vi "Wechart Get Token.vi"(8 "error in":errorcluster, 10 "appsecret":string="f200cec5fffa0616111cce48b6bc0b68", 11 "appID":string="wx6df44cfeabb6273b") -> (0 "error out":errorcluster, 3 "Token":string)   [LabVIEW 2020]
uses:
  <vilib>/httpClient/POSTBuffer.vi
  <vilib>/httpClient/LabVIEWHTTPClient.lvlib
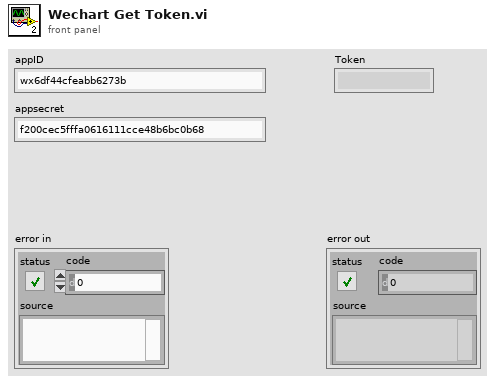
[diagram p1: front panel]
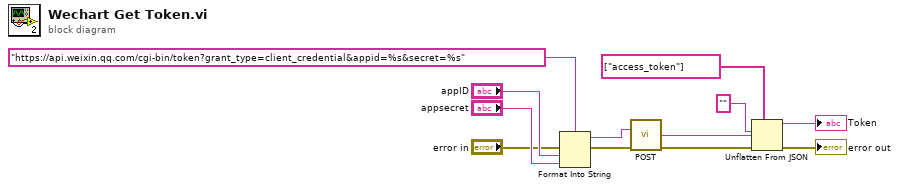
[diagram p0: block diagram]
diagram:
  n1 = Format Into String(format string="https://api.weixin.qq.com/cgi-bin/token?grant_type=client_credential&appid=%s&secret=%s" ("url"), error in="error in", "appID", "appsecret") -> (resulting string=w10:string, error out=w4:errorcluster)  [unwired: 1 in]
  n2 = call-poly <vilib>:"POST.vi"("url"=w10, "error in (no error)"=w4) -> ("body"=w9:string, "error out"=w3:errorcluster)  [unwired: 10 in, 2 out]
  n3 = Unflatten From JSON(path=string[] ["access_token"], JSON string=w9, type and defaults="", error in (no error)=w3) -> (value=→"Token":string, error out=→"error out":errorcluster)  [unwired: 3 in]
